vi "Ver 1.6.vi"() -> ()   [LabVIEW 2015]
uses:
  <instrlib>/Keithley 622x LV 2009/Configure/Source/Typedefs/KE622x -- Current Range.ctl
  <instrlib>/Keithley 622x LV 2009/Configure/Source/Typedefs/KE622x -- Current Ranges.ctl
  <instrlib>/Keithley 622x LV 2009/Typedefs/KE622x -- On Off Control.ctl
  <instrlib>/Keithley 622x LV 2009/Configure/Source/Typedefs/KE622x -- Voltage Limit.ctl
  <instrlib>/Keithley 622x LV 2009/Utility/Typedefs/KE622x -- Instrument Type.ctl
  <instrlib>/Keithley 2000/Public/Configure/Configure DC Volts.vi
  <userlib>/LV-Link3/PolySubVIs/DtCreateAinChan.vi
  <userlib>/LV-Link3/PolySubVIs/DtOLReadSingle.vi
  <instrlib>/Keithley 2000/Keithley 2000.lvlib
  <instrlib>/Keithley 622x LV 2009/Keithley 622x.lvlib
panel:
  out "5110":refnum<visa-resource-name>
  in  "GPIB Address":i8=12 min=1 max=32 step=1
  out "DAQ":dbl format="%#_13g"
  out "2000":dbl format="%#_13g"
  in  "Device":string(combo)
  in  "Channels":string="0"
  in  "Number \nof points":i32
  in  "Folder\nprename":string
  out "XY Graph":cluster{u32[], dbl[]}[](graph)
  out "T0":u32
  out "LIMIT":bool
  out "LIMIT":bool
  out "Error Code":string
  in  "Comments":string
  out "file":refnum<file>
  out "2000":refnum<visa-resource-name>
  out "6221":refnum<visa-resource-name>
  out "Step  (A)":dbl=5e-05 format="%#_3p"
  in  "Stop\ncurrent (A)":dbl=0.002 format="%#_6p"
  in  "Start \ncurrent (A)":dbl=0.001 format="%#_6p"
  in  "Check For SCPI Errors? (T)":bool=TRUE
  out "Interlock Tripped?":bool
  out "Compliance?":bool
  in  "Turn Off Output \nIf Compliance?":bool=TRUE
  in  "Turning ON/OFF\ncurrent output":T1=enum."On"
  in  "Range Selection":T2={"Auto Range?"=TRUE, "Man / Selected\nRange"=enum."2nA"}
  # "FILE CONFIGURATION"
  # "ADMIN PANEL"
  # "READINGS"
  # "KEITHLEY 6221 CONFIGURATION (ADMIN ONLY)"
  # "KEITHLEY DAQ CONFIGURATION (ADMIN ONLY)"
  # "PRINCETON LOCK-IN AMP (ADMIN ONLY)"
  # "I don't know what the hell it is,\njust don't touch it"
  # "START, STOP, STEP, CONFIGURATION"
  # "IF ON"
  # "Compliance = Limiting output voltage\nThis switch determines if we want to switch \noff the current output if wee exceed compliance"
  # "There is a safe switch at \nthe back of the instrument \nThis indicator shows if it is on"
  # "You have hit a damn jackpot \nby exceeding the limited voltage\nCongrats"
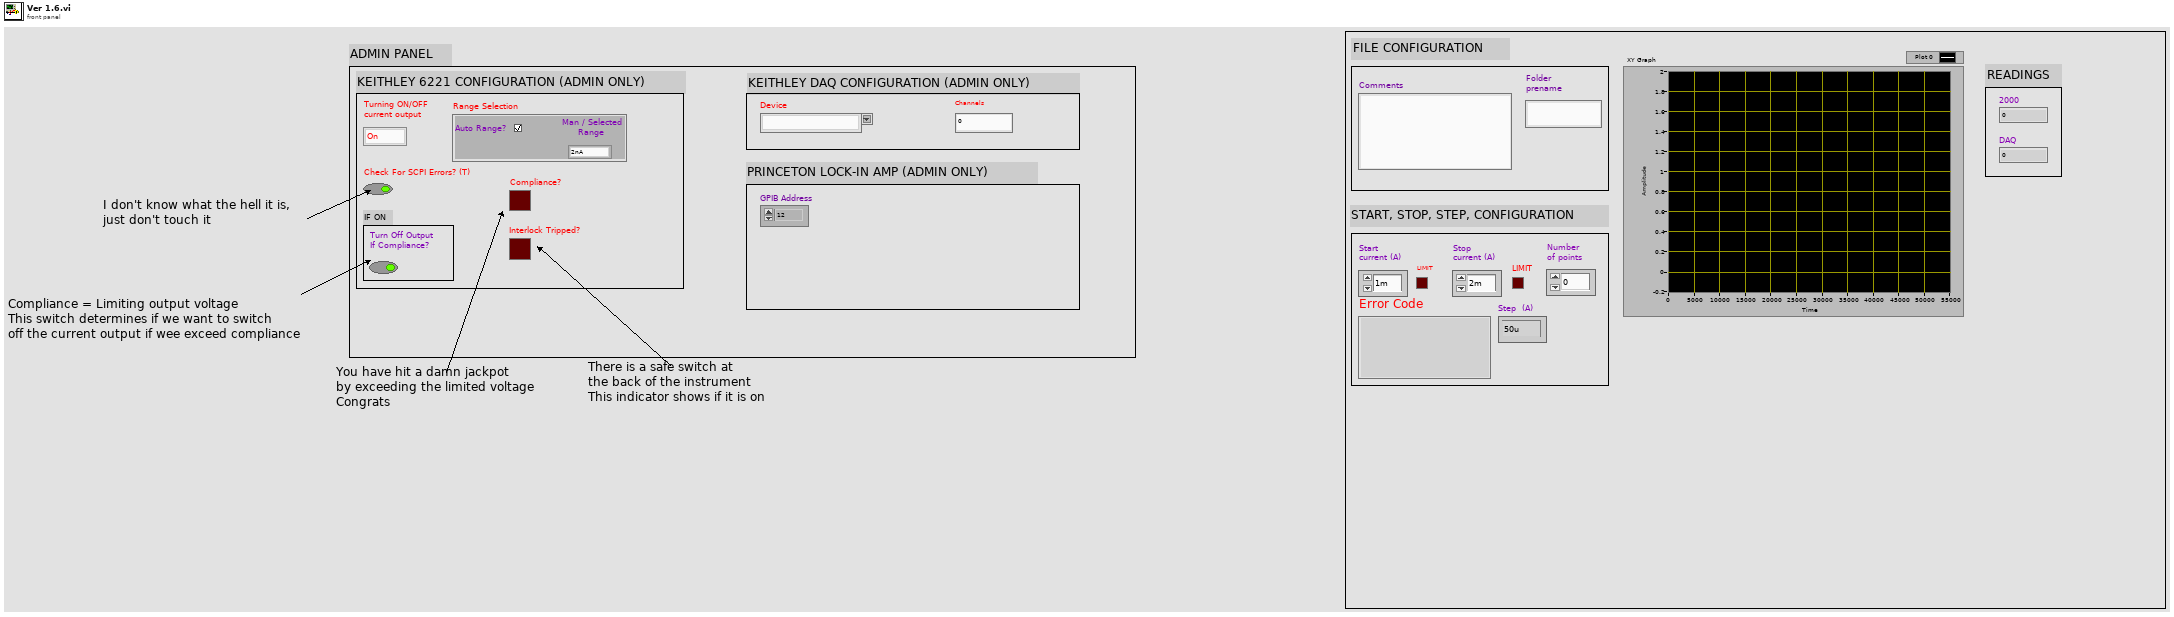
[diagram p1: front panel]
types:
  T1 = typedef "Keithley 622x.lvlib/KE622x -- On Off Control.ctl" = enum16{"Off", "On"}
  T2 = typedef "Keithley 622x.lvlib/KE622x -- Current Range.ctl" = cluster{"Auto Range?":bool, "Man / Selected\nRange":T3}
  T3 = typedef "Keithley 622x.lvlib/KE622x -- Current Ranges.ctl" = enum16{"2nA", "20nA", "200nA", "2uA", "20uA", "200uA", "2mA", "20mA", "100mA"}
  T4 = typedef "Keithley 622x.lvlib/KE622x -- Voltage Limit.ctl" = dbl
  T5 = typedef "Keithley 622x.lvlib/KE622x -- Instrument Type.ctl" = enum16{"KE6220", "KE6221"}
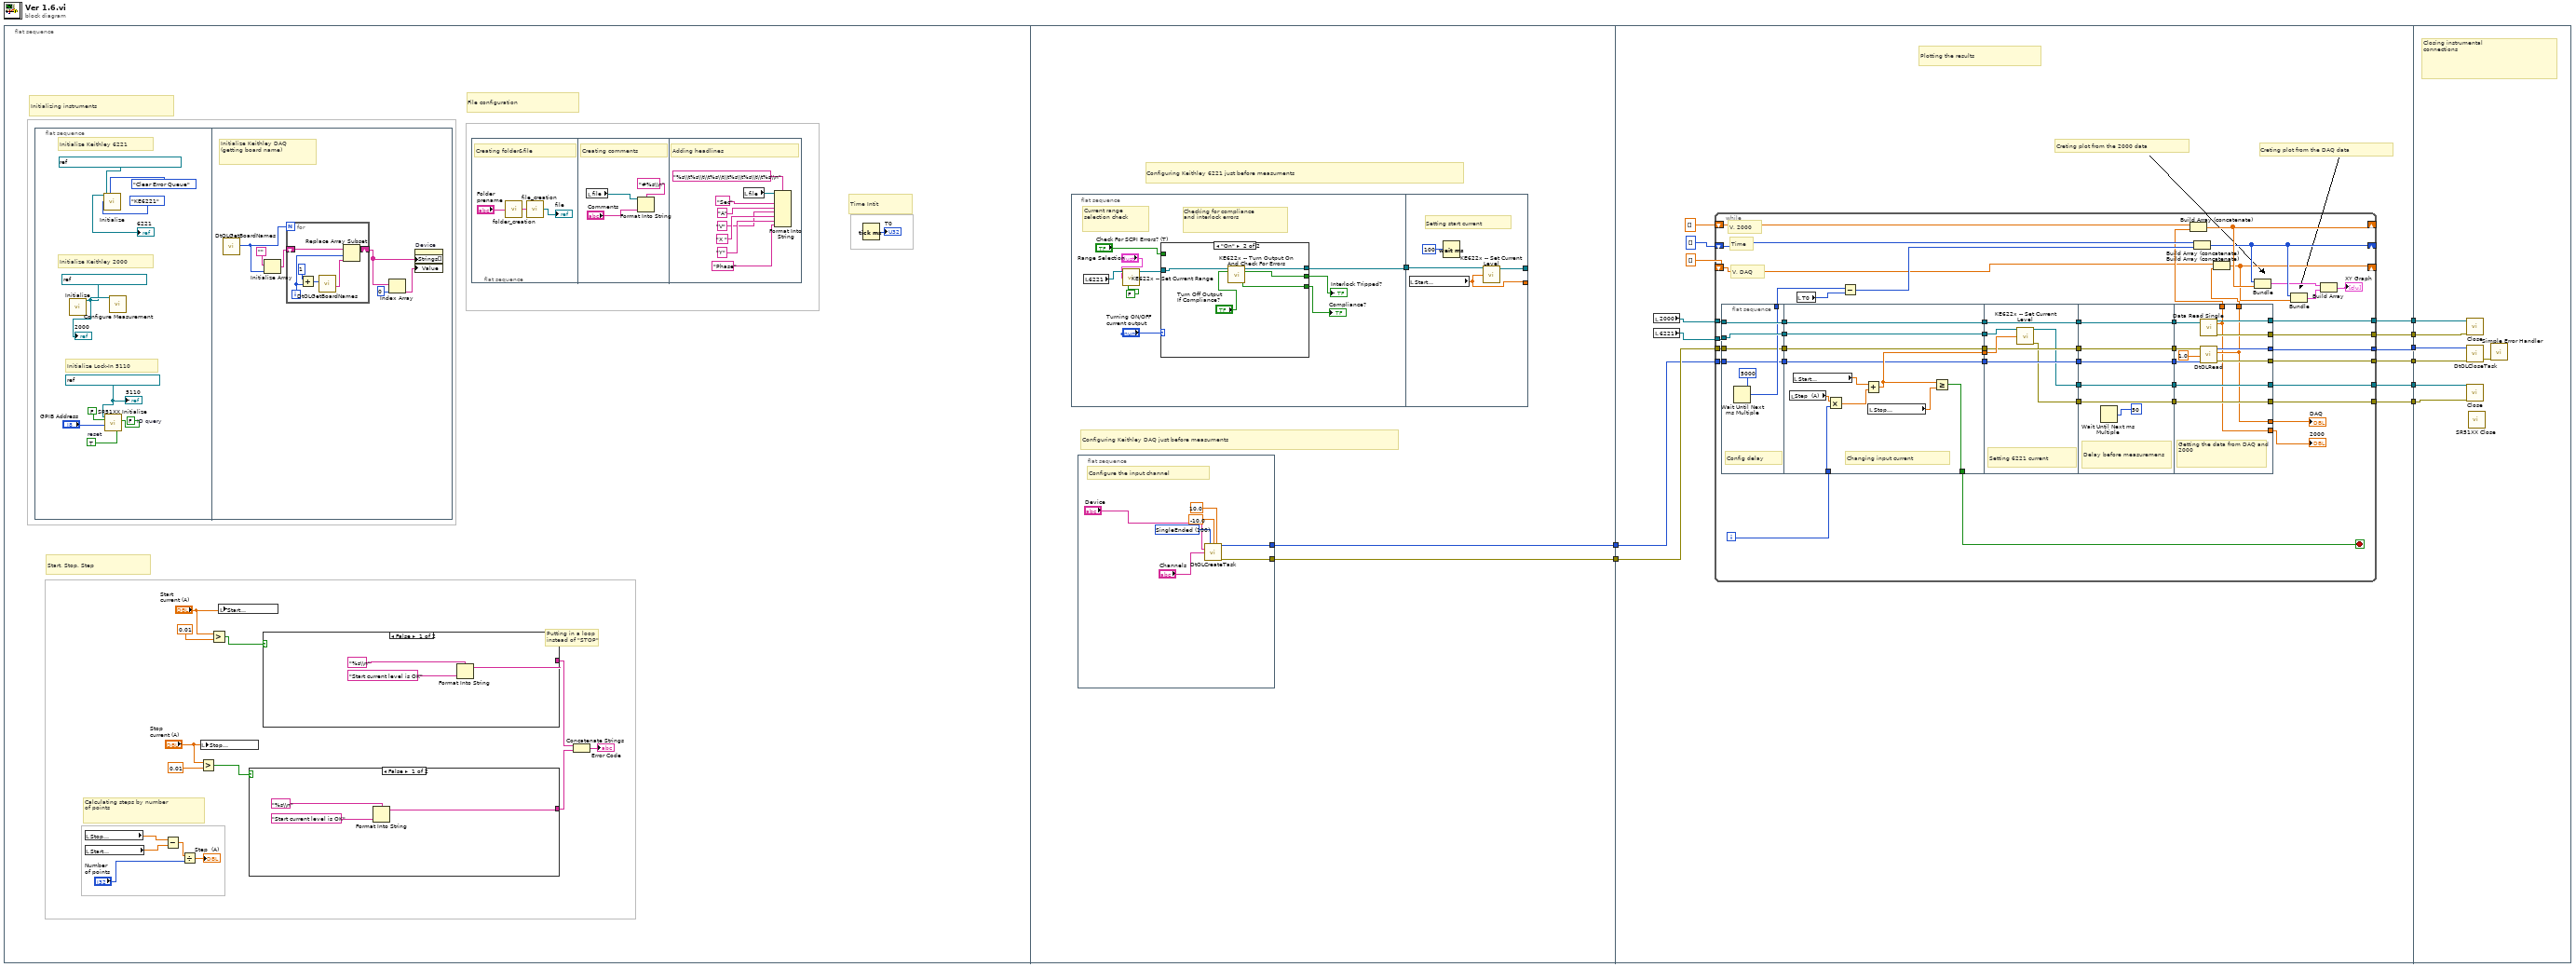
[diagram p0: block diagram]
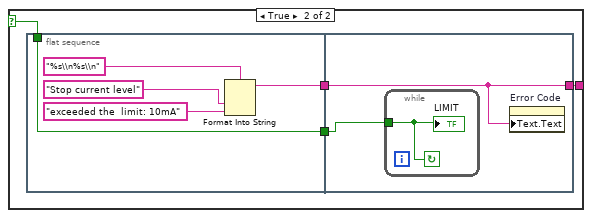
[diagram p2: hidden frame]
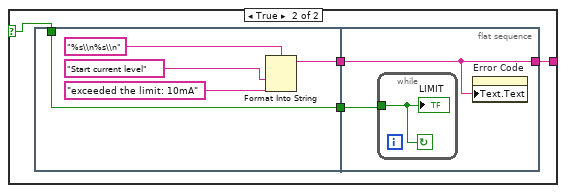
[diagram p3: hidden frame]
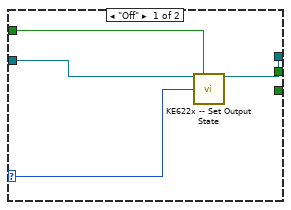
[diagram p4: hidden frame]
diagram:
  n1 = flat-sequence {
    tunnel: [w92] -> w8
    tunnel: [w91] -> w7
    tunnel: w8 -> [w132]
    tunnel: w7 -> [w133]
    tunnel: [w131] -> w6
    tunnel: [w129] -> w5
    tunnel: [w128] -> w4
    tunnel: [w127] -> w3
    tunnel: [w126] -> w2
    tunnel: [w125] -> w1
    tunnel: w6 -> [w230]
    tunnel: w5 -> [w229]
    tunnel: w4 -> [w228]
    tunnel: w3 -> [w227]
    tunnel: w2 -> [w226]
    tunnel: w1 -> [w225]
    frame #0 {
      # "Calculating steps by number\nof points"
      # "Time Intit"
      # "Putting in a loop \ninstead of \"STOP\""
      # "Start, Stop, Step"
      # "Initializing instruments"
      # "File configuration"
      n2 = flat-sequence {
        frame #0 {
          w24 = refnum<visa-resource-name> "LOCK_IN_5110_PRINCETON" ("VISA session (for class)")
          w26 = TRUE  # reset
          w25 = FALSE  # ID query
          # "Initialize Lock-In 5110"
          # "Initialize Keithley 2000"
          # "Initialize Keithley 6221"
          n3 = call <instrlib>:"Initialize.vi"("VISA resource name"=refnum<visa-resource-name> "KEITHLEY_MULTIMETER") -> ("VISA resource name out"=w30:refnum<visa-resource-name>)  [unwired: 17 in, 1 out]
          "2000" <- w30
          n4 = call <instrlib>:"Initialize.vi"("VISA resource name"=refnum<visa-resource-name> "KEITHLEY_DC_AC_CURRENT_SOURCE", "Error Queue Option"=enum16{"Clear Error Queue", "Error Query"}."Clear Error Queue", "Instrument Type"=KE622x_--_Instrument_Type."KE6221") -> ("VISA resource name out"=→"6221":refnum<visa-resource-name>)  [unwired: 11 in, 1 out]
          n5 = call "SR51XX Initialize"("VISA session (for class)"=w24, "Interface"=FALSE, "ID query"=w25, "GPIB Address"="GPIB Address", "reset"=w26) -> ()  [unwired: 8 in, 3 out]
          n6 = call-poly <instrlib>:"Configure Measurement.vi"("VISA resource name"=w30) -> ()  [unwired: 17 in, 2 out]
          "5110" <- w24
        }
        frame #1 {
          # "Initialize Keithley DAQ \n(getting board name)"
          n7 = call <userlib>:"DtOLGetBoardNames.vi"() -> ("Number of boards"=w35:u32)  [unwired: 9 in, 2 out]
          n8 = Initialize Array("", w35) -> (w37:string[])
          n9 = for {
            N: w35 -> [_]
            shift-right: [w43] -> w40
            shift-left: w37 -> [w44]
            i -> [w42]
            n10 = Add(x=1, y=w42) -> (x+y=w46:i32)
            n11 = call <userlib>:"DtOLGetBoardNames.vi"("Select Board"=w46) -> ("Board Name"=w41:string)  [unwired: 8 in, 2 out]
            n12 = Replace Array Subset(array=w44, new element=w41, index=w42) -> (w43:string[])
          }
          n13 = Index Array(array=w40, index=0) -> (element=w39:string)
          n14 = property on="Device" class="CmbBox"("Strings[]"=w40, "Value"=w39) -> ()  [unwired: 2 in, 2 out]
        }
      }
      n15 = local read "Stop\ncurrent (A)"() -> (w12:dbl)
      n16 = local read "Start \ncurrent (A)"() -> (w11:dbl)
      n17 = Subtract(x=w12, y=w11) -> (x-y=w9:dbl)
      n18 = Divide(x=w9, y="Number \nof points") -> (x/y=→"Step  (A)":dbl)
      n19 = Greater?(x="Stop\ncurrent (A)", y=T4 0.01) -> (0:w18:bool)
      n20 = local write "Stop\ncurrent (A)"("Stop\ncurrent (A)") -> ()
      n21 = Greater?(x="Start \ncurrent (A)", y=T4 0.01) -> (0:w19:bool)
      n22 = local write "Start \ncurrent (A)"("Start \ncurrent (A)") -> ()
      n23 = case shown="False" w18 {
        selector: w18 -> [_ w50]
        tunnel: [w47 w53] -> w16
        frame False {
          n24 = Format Into String(format string="%s\\n", "Start current level is OK" ("false string")) -> (resulting string=w47:string)  [unwired: 2 in, 1 out]
        }
        frame True {
          n25 = flat-sequence {
            tunnel: [w55] -> w52
            tunnel: [w54] -> w51
            tunnel: w50 -> [w54]
            tunnel: [w59] -> w53
            tunnel: w52 -> [w59]
            tunnel: w51 -> [w60]
            frame #0 {
              n26 = Format Into String(format string="%s\\n%s\\n", "Stop current level" ("String"), "exceeded the  limit: 10mA" ("input 2")) -> (resulting string=w55:string)  [unwired: 2 in, 1 out]
            }
            frame #1 {
              n27 = while {
                tunnel: w60 -> [w61]
                stop <- w61 continue-if-true
                "LIMIT" <- w61
              }
              n28 = property on="Error Code" class="Str"("Text.Text"=w59) -> ()  [unwired: 2 in, 2 out]
            }
          }
        }
      }
      n29 = case shown="False" w19 {
        selector: w19 -> [_ w66]
        tunnel: [w62 w68] -> w17
        frame False {
          n30 = Format Into String(format string="%s\\n", "Start current level is OK" ("false string")) -> (resulting string=w62:string)  [unwired: 2 in, 1 out]
        }
        frame True {
          n31 = flat-sequence {
            tunnel: [w70] -> w67
            tunnel: w66 -> [w69]
            tunnel: [w69] -> w65
            tunnel: [w74] -> w68
            tunnel: w67 -> [w74]
            tunnel: w65 -> [w75]
            frame #0 {
              n32 = Format Into String(format string="%s\\n%s\\n", "Start current level" ("String"), "exceeded the limit: 10mA" ("input 2")) -> (resulting string=w70:string)  [unwired: 2 in, 1 out]
            }
            frame #1 {
              n33 = while {
                tunnel: w75 -> [w76]
                stop <- w76 continue-if-true
                "LIMIT" <- w76
              }
              n34 = property on="Error Code" class="Str"("Text.Text"=w74) -> ()  [unwired: 2 in, 2 out]
            }
          }
        }
      }
      n35 = flat-sequence {
        frame #0 {
          # "Creating folder&file"
          n36 = call "folder_creation.vi"("Name"="Folder\nprename") -> ("String"=w78:string)
          n37 = call "file_creation.vi"("String"=w78) -> ("refnum out"=→"file":refnum<file>)
        }
        frame #1 {
          # "Creating comments"
          n38 = local read "file"() -> (w80:refnum<file>)
          n39 = Format Into String(format string="#%s\\n", initial string=w80, "Comments") -> ()  [unwired: 1 in, 2 out]
        }
        frame #2 {
          # "Adding headlines"
          n40 = local read "file"() -> (w90:refnum<file>)
          n41 = Format Into String(format string="%s\\t%s\\t\\t%s\\t\\t%s\\t%s\\t\\t%s\\n", initial string=w90, "Sec" ("input 1"), "A" ("input 2"), "V" ("input 3"), "X " ("input 3"), "Y" ("input 3"), "Phase" ("input 3")) -> ()  [unwired: 1 in, 2 out]
        }
      }
      n42 = Concatenate Strings(w17, w16) -> (→"Error Code":string)
      n43 = Tick Count (ms)() -> (millisecond timer value=→"T0":u32)
    }
    frame #1 {
      # "Configuring Keithley DAQ just before measuments"
      # "Configuring Keithley 6221 just before measuments"
      n44 = flat-sequence {
        tunnel: [w101] -> w93
        tunnel: [w119] -> _
        tunnel: [w121] -> _
        tunnel: w93 -> [w120]
        frame #0 {
          # "Current range \nselection check"
          # "Checking for compliance\nand interlock errors"
          n45 = local read "6221"() -> (w104:refnum<visa-resource-name>)
          n46 = call <instrlib>:"KE622x -- Set Current Range.vi"("Resource In"=w104, "Current Range In"="Range Selection", "Read Back Set Values? (T)"=FALSE) -> ("Resource Out (dupl)"=w109:refnum<visa-resource-name>)  [unwired: 10 in, 2 out]
          n47 = case shown="\"On\"" "Turning ON/OFF\ncurrent output" {
            selector: "Turning ON/OFF\ncurrent output" -> [w113 _]
            tunnel: [_ w117] -> w107
            tunnel: [_ w116] -> w108
            tunnel: "Check For SCPI Errors? (T)" -> [w112 _]
            tunnel: w109 -> [w110 w115]
            tunnel: [w111 w114] -> w101
            frame "Off" {
              n48 = call <instrlib>:"KE622x -- Set Output State.vi"("Resource In"=w110, "Check For SCPI Errors? (T)"=w112, "Output State"=w113) -> ("Resource Out (dupl)"=w111:refnum<visa-resource-name>)  [unwired: 11 in, 1 out]
            }
            frame "On" {
              n49 = call <instrlib>:"KE622x -- Turn Output On And Check For Errors.vi"("Resource In"=w115, "Turn Off Output If Compliance?"="Turn Off Output \nIf Compliance?") -> ("Resource Out (dupl)"=w114:refnum<visa-resource-name>, "Interlock Tripped?"=w117:bool, "Compliance?"=w116:bool)  [unwired: 10 in, 1 out]
            }
          }
          "Interlock Tripped?" <- w107
          "Compliance?" <- w108
        }
        frame #1 {
          # "Setting start current"
          n50 = local read "Start \ncurrent (A)"() -> (w119:dbl)
          n51 = Wait (ms)(milliseconds to wait=u32 100) -> ()  [unwired: 1 out]
          n52 = call <instrlib>:"KE622x -- Set Current Level.vi"("Resource In"=w120, "Current Level (A) In"=w119) -> ("Resource Out (dupl)"=w121:refnum<visa-resource-name>)  [unwired: 12 in, 1 out]
        }
      }
      n53 = flat-sequence {
        tunnel: [w95] -> w92
        tunnel: [w94] -> w91
        frame #0 {
          w99 = 100 items=["SingleEnded"=100, "Differential"=101] ("Channel Type")
          # "Configure the input channel"
          n54 = call-poly <userlib>:"DtOLCreateTask.vi"("Channel Type"=w99, "Range Min"=-10.0, "Range Max"=10.0, "Board Name"="Device", "Channel"="Channels") -> ("Task out"=w95:i32, "error out"=w94:errorcluster)  [unwired: 8 in, 1 out]
        }
      }
    }
    frame #2 {
      # "Plotting the results"
      # "Creting plot from the DAQ data"
      # "Creting plot from the 2000 data"
      n55 = local read "2000"() -> (w124:refnum<visa-resource-name>)
      n56 = local read "6221"() -> (w123:refnum<visa-resource-name>)
      n57 = while {
        shift-right: [w152] -> _
        shift-left: dbl[] [] -> [w182]
        shift-right: [w151] -> _
        shift-left: i32[] [] -> [w181]
        tunnel: w124 -> [w178]
        tunnel: w123 -> [w176]
        tunnel: w133 -> [w159]
        tunnel: w132 -> [w154]
        tunnel: [w165] -> w131
        shift-right: [w150] -> _
        shift-left: dbl[] [] -> [w164]
        tunnel: [w146] -> w129
        tunnel: [w145] -> w128
        tunnel: [w144] -> w127
        tunnel: [w142] -> w126
        tunnel: [w139] -> w125
        i -> [w172]
        stop <- w166 stop-if-true
        # "Time"
        # "V, DAQ"
        # "V, 2000"
        n58 = flat-sequence {
          tunnel: w178 -> [w188]
          tunnel: [w188] -> w177
          tunnel: w176 -> [w187]
          tunnel: [w187] -> w175
          tunnel: [w185] -> w174
          tunnel: [w184] -> w160
          tunnel: w159 -> [w184]
          tunnel: [w183] -> w155
          tunnel: w154 -> [w183]
          tunnel: [w199] -> w171
          tunnel: w177 -> [w199]
          tunnel: w175 -> [w194]
          tunnel: w172 -> [w196]
          tunnel: [w192] -> w166
          tunnel: [w191] -> w169
          tunnel: [w194] -> w168
          tunnel: [w190] -> w161
          tunnel: w160 -> [w190]
          tunnel: [w189] -> w156
          tunnel: w155 -> [w189]
          tunnel: w171 -> [w206]
          tunnel: [w206] -> w170
          tunnel: w169 -> [w205]
          tunnel: w168 -> [w204]
          tunnel: [w203] -> w162
          tunnel: w161 -> [w203]
          tunnel: [w202] -> w157
          tunnel: w156 -> [w202]
          tunnel: [w201] -> w143
          tunnel: [w200] -> w140
          tunnel: w170 -> [w212]
          tunnel: [w212] -> w173
          tunnel: [w210] -> w163
          tunnel: w162 -> [w210]
          tunnel: [w209] -> w158
          tunnel: w157 -> [w209]
          tunnel: w143 -> [w208]
          tunnel: [w208] -> w141
          tunnel: w140 -> [w207]
          tunnel: [w207] -> w138
          tunnel: w173 -> [w224]
          tunnel: [w213] -> w167
          tunnel: [w222] -> w165
          tunnel: w163 -> [w221]
          tunnel: w158 -> [w220]
          tunnel: [w214] -> w153
          tunnel: [w219] -> w146
          tunnel: [w218] -> w145
          tunnel: [w217] -> w144
          tunnel: [w216] -> w142
          tunnel: w141 -> [w216]
          tunnel: [w215] -> w139
          tunnel: w138 -> [w215]
          tunnel: [w214] -> w137
          tunnel: [w213] -> w136
          frame #0 {
            # "Config delay"
            n59 = Wait Until Next ms Multiple(millisecond multiple=u32 5000) -> (millisecond timer value=w185:u32)
          }
          frame #1 {
            # "Changing input current"
            n60 = local read "Step  (A)"() -> (w197:dbl)
            n61 = local read "Start \ncurrent (A)"() -> (w198:dbl)
            n62 = Multiply(x=w197, y=w196) -> (x*y=w195:dbl)
            n63 = Add(x=w198, y=w195) -> (x+y=w191:dbl)
            n64 = local read "Stop\ncurrent (A)"() -> (w193:dbl)
            n65 = Greater Or Equal?(x=w191, y=w193) -> (x >= y?=w192:bool)
          }
          frame #2 {
            # "Setting 6221 current"
            n66 = call <instrlib>:"KE622x -- Set Current Level.vi"("Resource In"=w204, "Current Level (A) In"=w205) -> ("Resource Out (dupl)"=w200:refnum<visa-resource-name>, "error out"=w201:errorcluster)  [unwired: 12 in]
          }
          frame #3 {
            # "Delay before measuremens"
            n67 = Wait Until Next ms Multiple(millisecond multiple=u32 50) -> ()  [unwired: 1 out]
          }
          frame #4 {
            # "Getting the data from DAQ and 2000"
            n68 = call-poly <userlib>:"DtOLRead.vi"("error in (no error)"=w221, "Timeout"=1.0, "Task in"=w220) -> ("error out"=w217:errorcluster, "Data Out"=w214:dbl, "Task out"=w222:i32)  [unwired: 6 in]
            n69 = call <instrlib>:"Data Read Single.vi"("VISA resource name"=w224) -> ("VISA resource name out"=w218:refnum<visa-resource-name>, "Measurement"=w213:dbl, "error out"=w219:errorcluster)  [unwired: 14 in, 2 out]
          }
        }
        n70 = local read "T0"() -> (w180:u32)
        n71 = Subtract(x=w174, y=w180) -> (x-y=w179:u32)
        n72 = Build Array (concatenate)(w182, w167) -> (w152:dbl[])
        n73 = Build Array (concatenate)(w181, w179) -> (w151:u32[])
        n74 = Build Array (concatenate)(w164, w153) -> (w150:dbl[])
        n75 = Bundle(w151, w152) -> (w148:cluster{u32[], dbl[]})  [unwired: 1 in]
        n76 = Bundle(w151, w150) -> (w147:cluster{u32[], dbl[]})  [unwired: 1 in]
        n77 = Build Array(w148, w147) -> (→"XY Graph":cluster{u32[], dbl[]}[])
        "2000" <- w136
        "DAQ" <- w137
      }
    }
    frame #3 {
      # "Closing instrumental \nconnections"
      n78 = call <instrlib>:"Close.vi"("VISA resource name"=w228, "error in (no error)"=w229) -> ()  [unwired: 17 in, 1 out]
      n79 = call <userlib>:"DtOLCloseTask.vi"("Error in"=w227, "Task in"=w230) -> ("Error Out"=w231:errorcluster)  [unwired: 9 in]
      n80 = call <instrlib>:"Close.vi"("VISA resource name"=w225, "error in (no error)"=w226) -> ()  [unwired: 13 in, 1 out]
      n81 = call "SR51XX Close"() -> ()  [unwired: 2 in, 1 out]
      n82 = call <vilib>:"Simple Error Handler.vi"("error in (no error)"=w231) -> ()  [unwired: 4 in, 5 out]
    }
  }
